vi "CRYChange Name Socket.vi"(9 "Data":string[][](array[string]), 10 "O_Signal Type":string[][](array[string]), 11 "I_Signal Type":string[][](array[string])) -> (3 "Changed Name":T1)   [LabVIEW 2013]
uses:
  CRYSystem/Typedef Control/CRYChanged Names Cluster.ctl
  CRYSystem/Typedef Control/CRYChanged Data Array Cluster.ctl
  CRYSystem/Typedef Control/CRYChanged Data Cluster.ctl
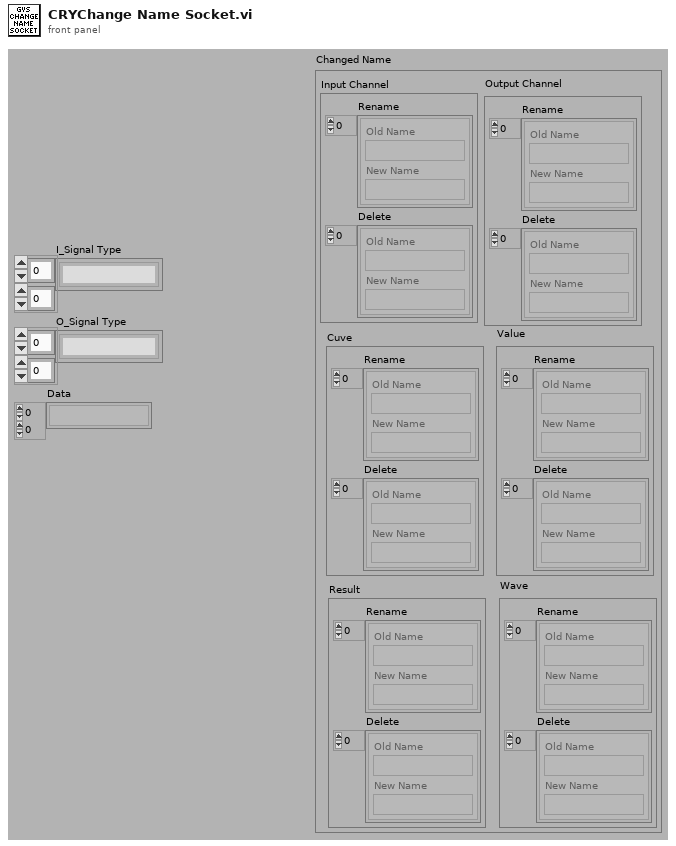
[diagram p1: front panel]
types:
  T1 = typedef "CRYChanged Names Cluster.ctl" = cluster{"Input Channel":T2, "Output Channel":T2, "Cuve":T2, "Value":T2, "Result":T2, "Wave":T2}
  T2 = typedef "CRYChanged Data Array Cluster.ctl" = cluster{"Rename":T3[], "Delete":T3[]}
  T3 = typedef "CRYChanged Data Cluster.ctl" = cluster{"Old Name":string, "New Name":string}
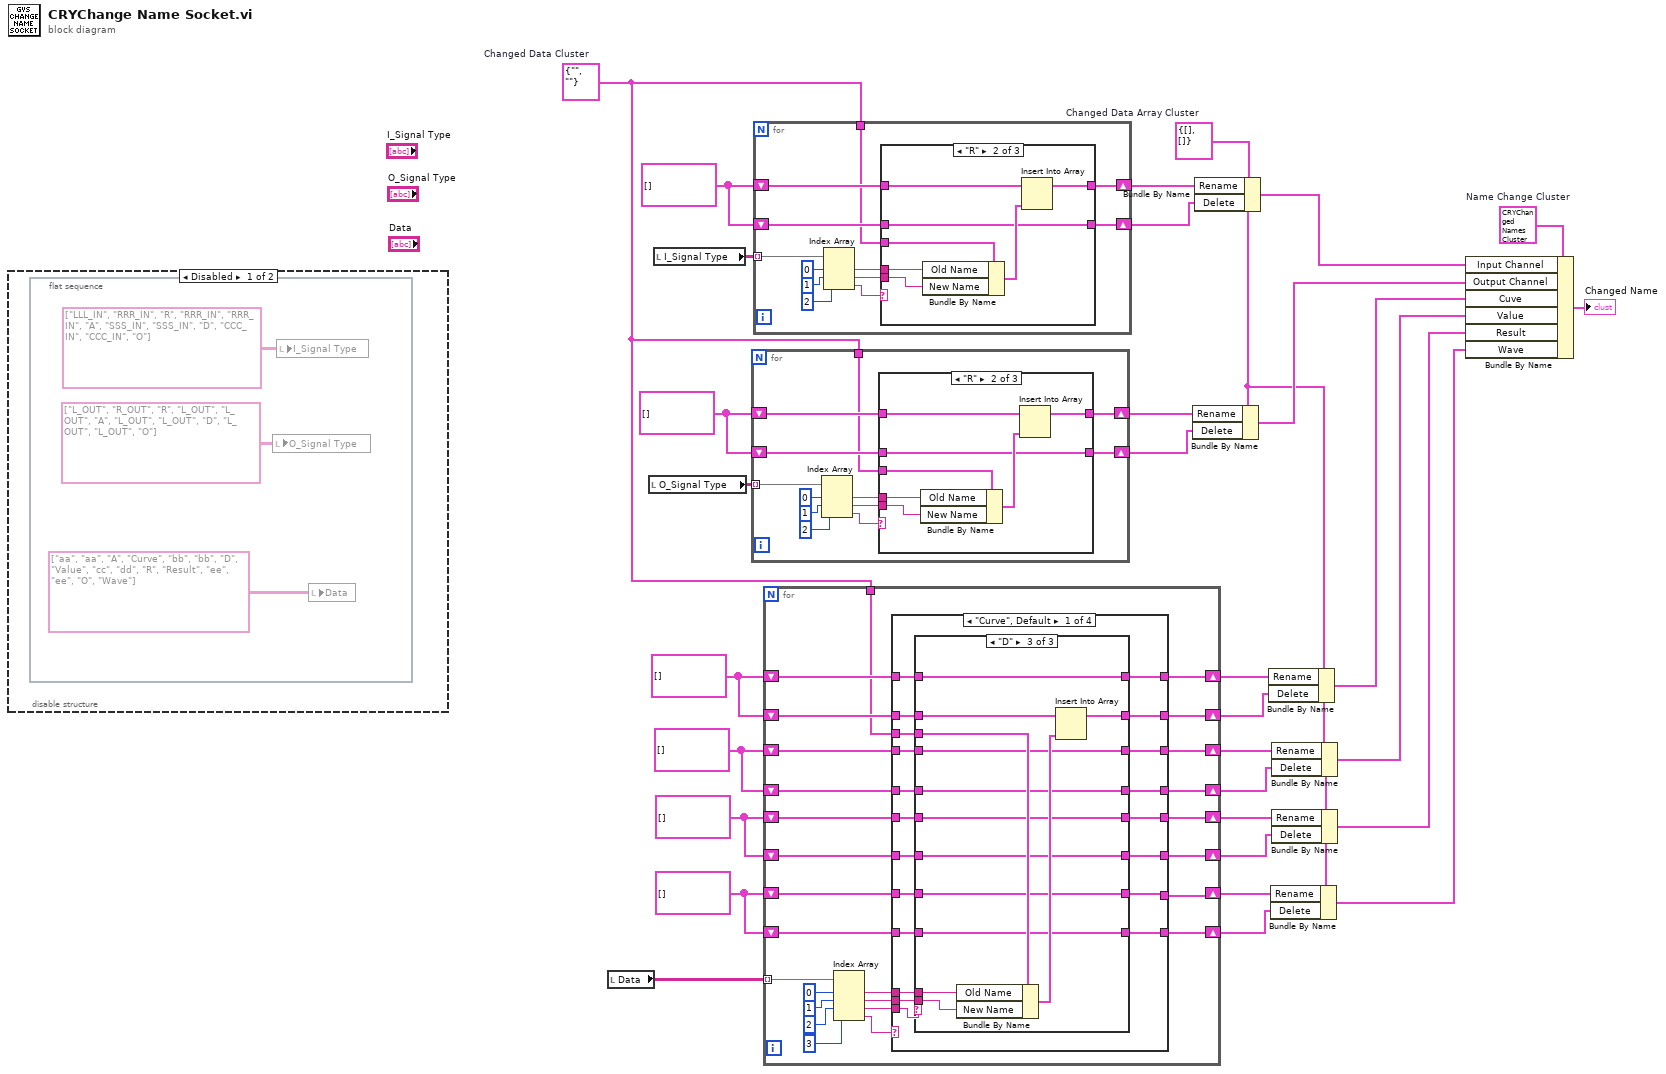
[diagram p0: block diagram]
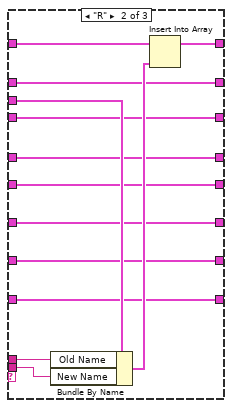
[diagram p4: hidden frame]
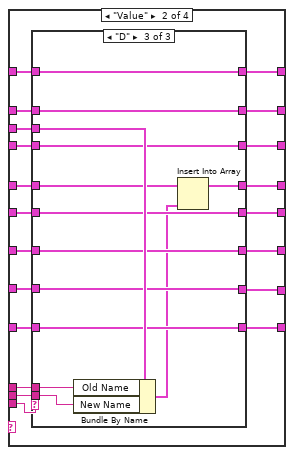
[diagram p5: hidden frame]
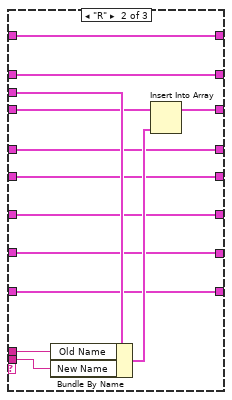
[diagram p7: hidden frame]
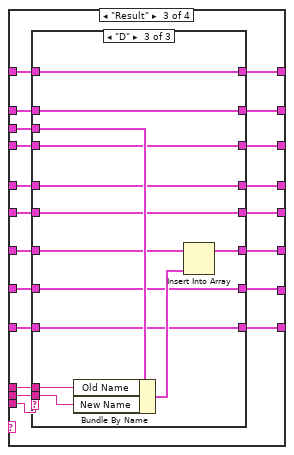
[diagram p8: hidden frame]
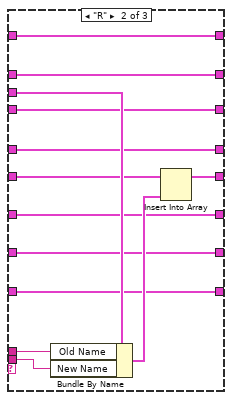
[diagram p10: hidden frame]
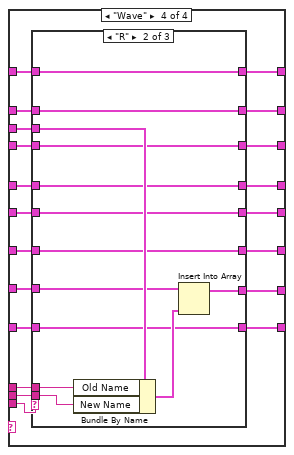
[diagram p11: hidden frame]
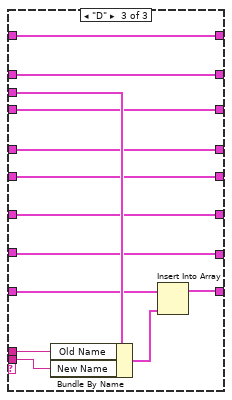
[diagram p13: hidden frame]
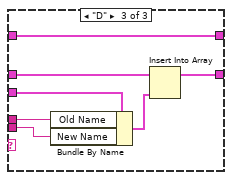
[diagram p15: hidden frame]
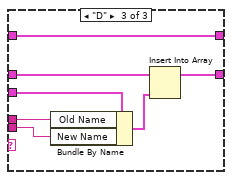
[diagram p17: hidden frame]
diagram:
  w1 = T2 {"Rename"=[], "Delete"=[]}  # Changed Data Array Cluster
  w12 = T3[] []
  w13 = T3[] []
  w14 = T3[] []
  w19 = T3[] []
  w22 = T3[] []
  w27 = T3[] []
  w15 = T3 {"Old Name"="", "New Name"=""}  # Changed Data Cluster
  w30 = T1 {"Input Channel"={"Rename"=[], "Delete"=[]}, "Output Channel"={"Rename"=[], "Delete"=[]}, "Cuve"={"Rename"=[], "Delete"=[]}, "Value"={"Rename"=[], "Delete"=[]}, "Result"={"Rename"=[], "Delete"=[]}, "Wave"={"Rename"=[], "Delete"=[]}}  # Name Change Cluster
  n1 = disable-structure shown="Disabled" {
    frame Disabled {
      n2 = flat-sequence {
        frame #0 {
          n3 = local write "O_Signal Type"(string[][] [["L_OUT", "R_OUT", "R"], ["L_OUT", "L_OUT", "A"], ["L_OUT", "L_OUT", "D"], ["L_OUT", "L_OUT", "O"]] ("O_Name In")) -> ()
          n4 = local write "I_Signal Type"(string[][] [["LLL_IN", "RRR_IN", "R"], ["RRR_IN", "RRR_IN", "A"], ["SSS_IN", "SSS_IN", "D"], ["CCC_IN", "CCC_IN", "O"]] ("I_Name In")) -> ()
          n5 = local write "Data"(string[][] [["aa", "aa", "A", "Curve"], ["bb", "bb", "D", "Value"], ["cc", "dd", "R", "Result"], ["ee", "ee", "O", "Wave"]] ("Calibration Data In")) -> ()
        }
      }
    }
    frame Enabled {
    }
  }
  n6 = local read "Data"() -> (w16:string[][])
  n7 = local read "O_Signal Type"() -> (w21:string[][])
  n8 = local read "I_Signal Type"() -> (w31:string[][])
  n9 = for {
    tunnel: w21 -> [w45] mode=indexing
    shift-right: [w35] -> w23
    shift-left: w22 -> [w39]
    shift-right: [w36] -> w24
    shift-left: w22 -> [w38]
    tunnel: w15 -> [w37]
    n10 = Index Array(array=w45, index #1=0 ("index"), index #2=1 ("index"), index #3=2 ("index")) -> (element #1=w41:string, element #2=w42:string, element #3=w40:string)
    n11 = case shown="\"R\"" w40 {
      tunnel: w42 -> [_ w55 w62]
      tunnel: w41 -> [_ w54 w61]
      tunnel: [w47 w49 w60] -> w36
      tunnel: w39 -> [w48 w53 w56]
      tunnel: w38 -> [w47 w49 w57]
      tunnel: w37 -> [_ w51 w58]
      tunnel: [w48 w50 w56] -> w35
      frame "A", "O", Default {
      }
      frame "R" {
        n12 = Bundle By Name(cluster=w51, "Old Name"=w54, "New Name"=w55) -> (w52:T3)
        n13 = Insert Into Array(array=w53, new element=w52) -> (w50:T3[])  [unwired: 1 in]
      }
      frame "D" {
        n14 = Bundle By Name(cluster=w58, "Old Name"=w61, "New Name"=w62) -> (w59:T3)
        n15 = Insert Into Array(array=w57, new element=w59) -> (w60:T3[])  [unwired: 1 in]
      }
    }
  }
  n16 = for {
    tunnel: w31 -> [w73] mode=indexing
    shift-right: [w63] -> w26
    shift-left: w27 -> [w67]
    shift-right: [w64] -> w25
    shift-left: w27 -> [w66]
    tunnel: w15 -> [w65]
    n17 = Index Array(array=w73, index #1=0 ("index"), index #2=1 ("index"), index #3=2 ("index")) -> (element #1=w69:string, element #2=w70:string, element #3=w68:string)
    n18 = case shown="\"R\"" w68 {
      tunnel: w70 -> [_ w83 w90]
      tunnel: w69 -> [_ w82 w89]
      tunnel: [w75 w77 w88] -> w64
      tunnel: w67 -> [w76 w81 w84]
      tunnel: w66 -> [w75 w77 w85]
      tunnel: w65 -> [_ w79 w86]
      tunnel: [w76 w78 w84] -> w63
      frame "A", "O", Default {
      }
      frame "R" {
        n19 = Bundle By Name(cluster=w79, "Old Name"=w82, "New Name"=w83) -> (w80:T3)
        n20 = Insert Into Array(array=w81, new element=w80) -> (w78:T3[])  [unwired: 1 in]
      }
      frame "D" {
        n21 = Bundle By Name(cluster=w86, "Old Name"=w89, "New Name"=w90) -> (w87:T3)
        n22 = Insert Into Array(array=w85, new element=w87) -> (w88:T3[])  [unwired: 1 in]
      }
    }
  }
  n23 = for {
    tunnel: w16 -> [w115] mode=indexing
    shift-right: [w105] -> w18
    shift-left: w19 -> [w109]
    shift-right: [w106] -> w17
    shift-left: w19 -> [w108]
    tunnel: w15 -> [w107]
    shift-right: [w101] -> w11
    shift-left: w14 -> [w102]
    shift-right: [w99] -> w10
    shift-left: w14 -> [w100]
    shift-right: [w97] -> w9
    shift-left: w13 -> [w98]
    shift-right: [w96] -> w8
    shift-left: w13 -> [w95]
    shift-right: [w93] -> w7
    shift-left: w12 -> [w94]
    shift-right: [w92] -> w6
    shift-left: w12 -> [w91]
    n24 = Index Array(array=w115, index #1=0 ("index"), index #2=1 ("index"), index #3=2 ("index"), index #4=3 ("index")) -> (element #1=w111:string, element #2=w112:string, element #3=w110:string, element #4=w103:string)
    n25 = case shown="\"Curve\", Default" w103 {
      tunnel: w112 -> [w136 w190 w244 w298]
      tunnel: w111 -> [w135 w189 w243 w297]
      tunnel: w110 -> [w134 w188 w242 w296]
      tunnel: w109 -> [w133 w187 w241 w295]
      tunnel: w108 -> [w132 w186 w240 w294]
      tunnel: w107 -> [w131 w185 w239 w293]
      tunnel: [w130 w184 w238 w292] -> w106
      tunnel: [w129 w183 w237 w291] -> w105
      tunnel: w102 -> [w127 w182 w235 w285]
      tunnel: [w128 w181 w236 w286] -> w101
      tunnel: w100 -> [w125 w180 w233 w283]
      tunnel: [w126 w179 w234 w284] -> w99
      tunnel: w98 -> [w123 w177 w232 w281]
      tunnel: [w124 w178 w231 w282] -> w97
      tunnel: [w122 w176 w230 w280] -> w96
      tunnel: w95 -> [w121 w175 w229 w279]
      tunnel: w94 -> [w117 w173 w227 w290]
      tunnel: [w118 w174 w228 w289] -> w93
      tunnel: [w120 w172 w226 w288] -> w92
      tunnel: w91 -> [w119 w171 w225 w287]
      frame "Curve", Default {
        n26 = case shown="\"D\"" w134 {
          tunnel: w136 -> [_ w157 w170]
          tunnel: w135 -> [_ w156 w169]
          tunnel: [w143 w151 w168] -> w130
          tunnel: w133 -> [w144 w155 w164]
          tunnel: w132 -> [w143 w151 w165]
          tunnel: w131 -> [_ w153 w166]
          tunnel: [w144 w152 w164] -> w129
          tunnel: [w142 w150 w163] -> w128
          tunnel: w127 -> [w142 w150 w163]
          tunnel: [w141 w149 w162] -> w126
          tunnel: w125 -> [w141 w149 w162]
          tunnel: [w140 w148 w161] -> w124
          tunnel: w123 -> [w140 w148 w161]
          tunnel: [w139 w147 w160] -> w122
          tunnel: w121 -> [w139 w147 w160]
          tunnel: [w137 w146 w158] -> w120
          tunnel: w119 -> [w137 w146 w158]
          tunnel: [w138 w145 w159] -> w118
          tunnel: w117 -> [w138 w145 w159]
          frame "A", "O", Default {
          }
          frame "R" {
            n27 = Bundle By Name(cluster=w153, "Old Name"=w156, "New Name"=w157) -> (w154:T3)
            n28 = Insert Into Array(array=w155, new element=w154) -> (w152:T3[])  [unwired: 1 in]
          }
          frame "D" {
            n29 = Bundle By Name(cluster=w166, "Old Name"=w169, "New Name"=w170) -> (w167:T3)
            n30 = Insert Into Array(array=w165, new element=w167) -> (w168:T3[])  [unwired: 1 in]
          }
        }
      }
      frame "Value" {
        n31 = case shown="\"D\"" w188 {
          tunnel: w190 -> [_ w211 w224]
          tunnel: w189 -> [_ w210 w223]
          tunnel: [w197 w208 w221] -> w184
          tunnel: w187 -> [w198 w207 w220]
          tunnel: w186 -> [w197 w208 w221]
          tunnel: w185 -> [_ w209 w222]
          tunnel: [w198 w207 w220] -> w183
          tunnel: w182 -> [w196 w206 w219]
          tunnel: [w196 w205 w219] -> w181
          tunnel: w180 -> [w195 w203 w213]
          tunnel: [w195 w203 w212] -> w179
          tunnel: [w194 w202 w215] -> w178
          tunnel: w177 -> [w194 w202 w215]
          tunnel: [w193 w201 w218] -> w176
          tunnel: w175 -> [w193 w201 w218]
          tunnel: [w192 w200 w217] -> w174
          tunnel: w173 -> [w192 w200 w217]
          tunnel: [w191 w199 w216] -> w172
          tunnel: w171 -> [w191 w199 w216]
          frame "A", "O", Default {
          }
          frame "R" {
            n32 = Bundle By Name(cluster=w209, "Old Name"=w210, "New Name"=w211) -> (w204:T3)
            n33 = Insert Into Array(array=w206, new element=w204) -> (w205:T3[])  [unwired: 1 in]
          }
          frame "D" {
            n34 = Bundle By Name(cluster=w222, "Old Name"=w223, "New Name"=w224) -> (w214:T3)
            n35 = Insert Into Array(array=w213, new element=w214) -> (w212:T3[])  [unwired: 1 in]
          }
        }
      }
      frame "Result" {
        n36 = case shown="\"D\"" w242 {
          tunnel: w244 -> [_ w265 w278]
          tunnel: w243 -> [_ w264 w277]
          tunnel: [w251 w262 w275] -> w238
          tunnel: w241 -> [w252 w261 w274]
          tunnel: w240 -> [w251 w262 w275]
          tunnel: w239 -> [_ w263 w276]
          tunnel: [w252 w261 w274] -> w237
          tunnel: [w250 w260 w273] -> w236
          tunnel: w235 -> [w250 w260 w273]
          tunnel: [w249 w259 w272] -> w234
          tunnel: w233 -> [w249 w259 w272]
          tunnel: w232 -> [w248 w257 w271]
          tunnel: [w248 w256 w271] -> w231
          tunnel: [w247 w255 w269] -> w230
          tunnel: w229 -> [w247 w255 w268]
          tunnel: [w246 w254 w267] -> w228
          tunnel: w227 -> [w246 w254 w267]
          tunnel: [w245 w253 w266] -> w226
          tunnel: w225 -> [w245 w253 w266]
          frame "A", "O", Default {
          }
          frame "R" {
            n37 = Bundle By Name(cluster=w263, "Old Name"=w264, "New Name"=w265) -> (w258:T3)
            n38 = Insert Into Array(array=w257, new element=w258) -> (w256:T3[])  [unwired: 1 in]
          }
          frame "D" {
            n39 = Bundle By Name(cluster=w276, "Old Name"=w277, "New Name"=w278) -> (w270:T3)
            n40 = Insert Into Array(array=w268, new element=w270) -> (w269:T3[])  [unwired: 1 in]
          }
        }
      }
      frame "Wave" {
        n41 = case shown="\"R\"" w296 {
          tunnel: w298 -> [_ w319 w332]
          tunnel: w297 -> [_ w318 w331]
          tunnel: [w305 w316 w329] -> w292
          tunnel: w295 -> [w306 w311 w328]
          tunnel: w294 -> [w305 w316 w329]
          tunnel: w293 -> [_ w317 w330]
          tunnel: [w306 w311 w328] -> w291
          tunnel: w290 -> [w300 w315 w323]
          tunnel: [w300 w314 w323] -> w289
          tunnel: [w299 w312 w320] -> w288
          tunnel: w287 -> [w299 w312 w321]
          tunnel: [w304 w310 w327] -> w286
          tunnel: w285 -> [w304 w310 w327]
          tunnel: [w303 w309 w326] -> w284
          tunnel: w283 -> [w303 w309 w326]
          tunnel: [w302 w308 w325] -> w282
          tunnel: w281 -> [w302 w308 w325]
          tunnel: [w301 w307 w324] -> w280
          tunnel: w279 -> [w301 w307 w324]
          frame "A", "O", Default {
          }
          frame "R" {
            n42 = Bundle By Name(cluster=w317, "Old Name"=w318, "New Name"=w319) -> (w313:T3)
            n43 = Insert Into Array(array=w315, new element=w313) -> (w314:T3[])  [unwired: 1 in]
          }
          frame "D" {
            n44 = Bundle By Name(cluster=w330, "Old Name"=w331, "New Name"=w332) -> (w322:T3)
            n45 = Insert Into Array(array=w321, new element=w322) -> (w320:T3[])  [unwired: 1 in]
          }
        }
      }
    }
  }
  n46 = Bundle By Name(cluster=w1, "Rename"=w23, "Delete"=w24) -> (w20:T2)
  n47 = Bundle By Name(cluster=w1, "Rename"=w26, "Delete"=w25) -> (w28:T2)
  n48 = Bundle By Name(cluster=w1, "Rename"=w18, "Delete"=w17) -> (w5:T2)
  n49 = Bundle By Name(cluster=w1, "Rename"=w7, "Delete"=w6) -> (w2:T2)
  n50 = Bundle By Name(cluster=w1, "Rename"=w11, "Delete"=w10) -> (w4:T2)
  n51 = Bundle By Name(cluster=w1, "Rename"=w9, "Delete"=w8) -> (w3:T2)
  n52 = Bundle By Name(cluster=w30, "Input Channel"=w28, "Output Channel"=w20, "Cuve"=w5, "Value"=w4, "Result"=w3, "Wave"=w2) -> (→"Changed Name":T1)
